vi "Write Status.vi"(8 "error in (no error)":errorcluster, 10 "Status":bool, 11 "SciShutt in":refnum<class "SciShutt.lvclass">) -> (0 "error out":errorcluster, 3 "SciShutt out":refnum<class "SciShutt.lvclass">)   [LabVIEW 2016, in "SciShutt.lvclass"]
uses:
  SciShutt.lvclass
  BiStable/BiStableShutter.lvclass
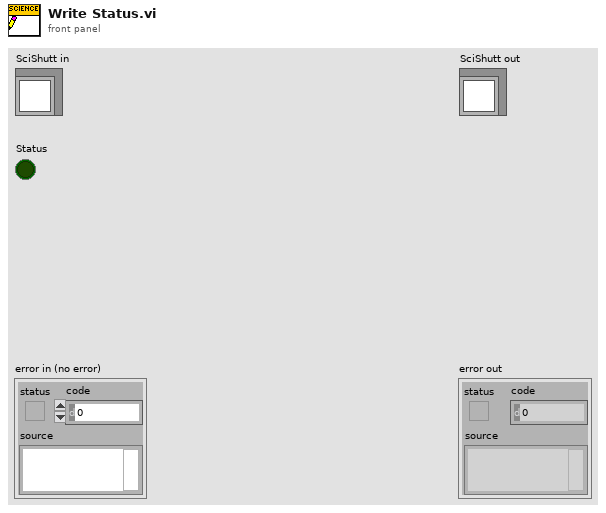
[diagram p1: front panel]
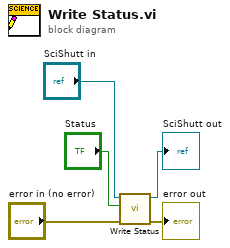
[diagram p0: block diagram]
diagram:
  n1 = call-parent "Write Status.vi"("error in (no error)"="error in (no error)", "Status"="Status", "Shutter in"="SciShutt in") -> ("error out"=→"error out":errorcluster, "Shutter out"=→"SciShutt out":refnum<class "SciShutt.lvclass">)  [unwired: 7 in]
